vi "get_level.vi"(8 "error in (no error)":errorcluster, 11 "NIErrLog Log Provider in":refnum<class "NIErrLog Log Provider.lvclass">) -> (0 "error out":errorcluster, 1 "level":T1 items=["OFF"=0, "FATAL"=100, "ERROR"=200, "WARN"=300, "INFO"=400, "DEBUG"=500, "TRACE"=600, "ALL"=65535], 3 "NIErrLog Log Provider out":refnum<class "NIErrLog Log Provider.lvclass">)   [LabVIEW 2019, in "NIErrLog Log Provider.lvclass"]
uses:
  NIErrLog Log Provider.lvclass
  Log Service/public/level.ctl
  NIErrLog Log Provider.lvclass/NIErrLog Log Provider.ctl
  Log Service/Log Service.lvclass
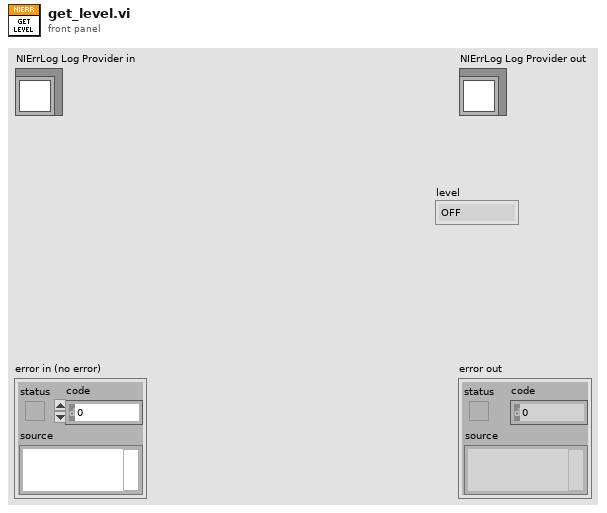
[diagram p1: front panel]
types:
  T1 = typedef "Utility API.lvlib/Log Service.lvclass/level.ctl" = u16
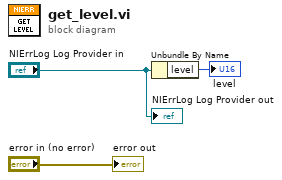
[diagram p0: block diagram]
diagram:
  n1 = Unbundle By Name("NIErrLog Log Provider in") -> ("level"=→"level":T1)
  "error out" <- "error in (no error)"
  "NIErrLog Log Provider out" <- "NIErrLog Log Provider in"
